vi "Angle Converter- Unit Circle Radians to Degrees.vi"(11 "Angle in \nUnit Circle\nRadians":dbl) -> (3 "Angle in \nHeading \nFormat":T1 format="%05.1f")   [LabVIEW 2011]
doc: "Converts angles in heading format (clockwise degrees with North = 0) to unit circle radians (counterclockwise, East = positive X direction = 0)\nUse this before applying trigonometric functions to headings."
uses:
  2 Typedefs/heading.ctl
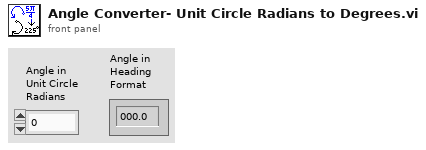
[diagram p1: front panel]
types:
  T1 = typedef "heading.ctl" = dbl
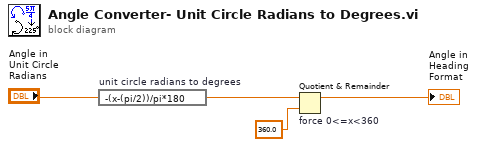
[diagram p0: block diagram]
diagram:
  n1 = expression code="-(x-(pi/2))/pi*180" "unit circle radians to degrees"("Angle in \nUnit Circle\nRadians") -> (w2:dbl)
  n2 = Quotient & Remainder "force 0<=x<360"(x=w2, y=360.0) -> (x-y*floor(x/y)=→"Angle in \nHeading \nFormat":dbl)  [unwired: 1 out]
